vi "controlGenerator.vi"(8 "error in (no error)":errorcluster, 10 "ControlOutputPath":path, 11 "ComponentIDLFile":path) -> (0 "error out":errorcluster)   [LabVIEW 2018]
uses:
  IDLFile/IDLFile.lvclass
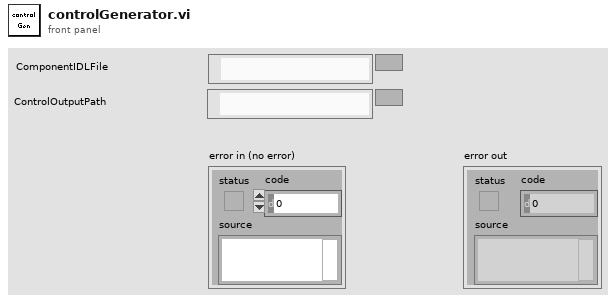
[diagram p1: front panel]
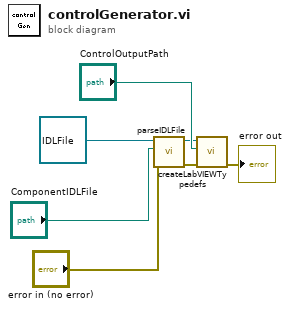
[diagram p0: block diagram]
diagram:
  n1 = call "parseIDLFile.vi"("error in (no error)"="error in (no error)", "idlFilepath"="ComponentIDLFile", "IDLFile in"=refnum<class "IDLFile.lvclass"> refnum ("IDLParser in")) -> ("error out"=w3:errorcluster, "IDLFile out"=w4:refnum<class "IDLFile.lvclass">)  [unwired: 7 in]
  n2 = call "createLabVIEWTypedefs.vi"("error in (no error)"=w3, "targetBasePath"="ControlOutputPath", "IDLFile in"=w4) -> ("error out"=→"error out":errorcluster)  [unwired: 7 in, 1 out]
